vi "saveInstrumentScript.vi"(6 "scriptName":string, 8 "error in (no error)":errorcluster, 9 "timeStamp":string, 10 "folderPath":path, 11 "device in":refnum<class "device.lvclass">) -> (0 "error out":errorcluster, 3 "device out":refnum<class "device.lvclass">)   [LabVIEW 2011, in "Tools.lvlib" / "DatabaseHelpers.lvlib" / "device.lvclass"]
uses:
  device.lvclass
  XmlParser.lvclass
  device.lvclass/device.ctl
  xmlNode/xmlNode.lvclass
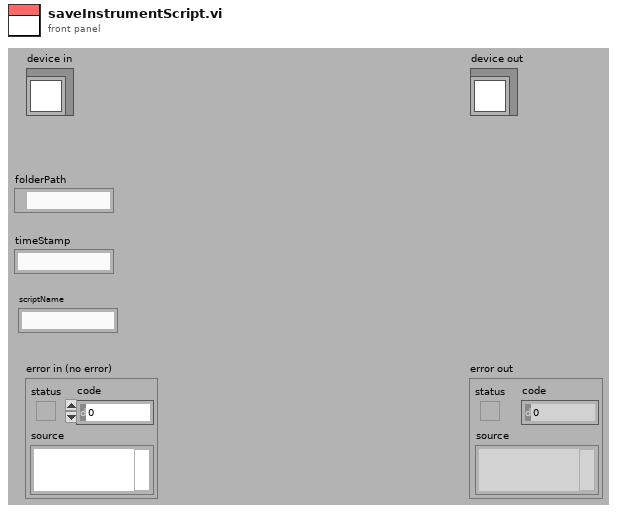
[diagram p1: front panel]
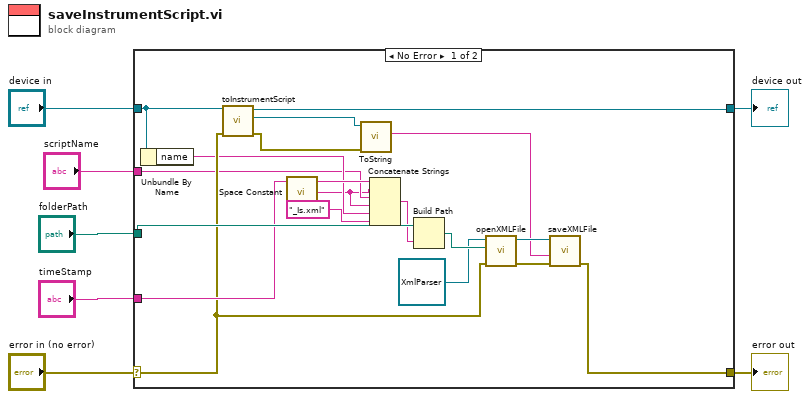
[diagram p0: block diagram]
diagram:
  n1 = case shown="No Error" "error in (no error)" {
    selector: "error in (no error)" -> [w19 w27]
    tunnel: [w12 w27] -> w6
    tunnel: [w25 w26] -> w4
    tunnel: "device in" -> [w23 w26]
    tunnel: "folderPath" -> [w24 _]
    tunnel: "timeStamp" -> [w22 _]
    tunnel: "scriptName" -> [w9 _]
    frame No Error {
      n2 = Unbundle By Name(w23) -> ("name"=w11:string)
      n3 = call-dynamic "toInstrumentScript.vi"("error in (no error)"=w19, "device in"=w23) -> ("error out"=w14:errorcluster, "instrument_ScriptXml"=w15:refnum<class "xmlNode.lvclass">, "device out"=w25:refnum<class "device.lvclass">)  [unwired: 7 in]
      n4 = call <vilib>:"Space Constant.vi"() -> ("String"=w8:string)
      n5 = call-dynamic "ToString.vi"("error in (no error)"=w14, "xmlNode in"=w15) -> ("xml"=w13:string)  [unwired: 7 in, 2 out]
      n6 = Concatenate Strings(w22, w8, w9, w8, w11, "_Is.xml") -> (w21:string)
      n7 = Build Path(base path=w24, name or relative path=w21) -> (appended path=w20:path)
      n8 = call "openXMLFile.vi"("error in (no error)"=w19, "Path"=w20, "XmlParser in"=refnum<class "XmlParser.lvclass"> refnum) -> ("error out"=w17:errorcluster, "XmlParser out"=w16:refnum<class "XmlParser.lvclass">)  [unwired: 6 in, 1 out]
      n9 = call-dynamic "saveXMLFile.vi"("error in (no error)"=w17, "xmlString"=w13, "XmlParser in"=w16) -> ("error out"=w12:errorcluster)  [unwired: 7 in, 1 out]
    }
    frame Error {
    }
  }
  "error out" <- w6
  "device out" <- w4
